vi "LoopselFF.VI"() -> ()   [LabVIEW 2015]
panel:
  in  "pos slope":u8=1
  in  "both slopes":u8
  in  "block Trig 0/1":u8
  in  "DAT in 10ns":u32
  out "FIFO overflow":bool
  in  "extTrig 0/1":u8
  in  "stop all":bool
  in  "Arm/Clear arry":bool
  in  "Slide":u32(slide)=1 scale=1.0..1000.0
  in  "frequency[Hz]":u32
  in  "no.of samples (nos)":u32=1000
  in  "exposuretime[ms]":dbl=0.02 format="%.3f"
  out "Signalverlaufgraph":u16[](graph)
  # "Abort with ESC"
  # "Start with run"
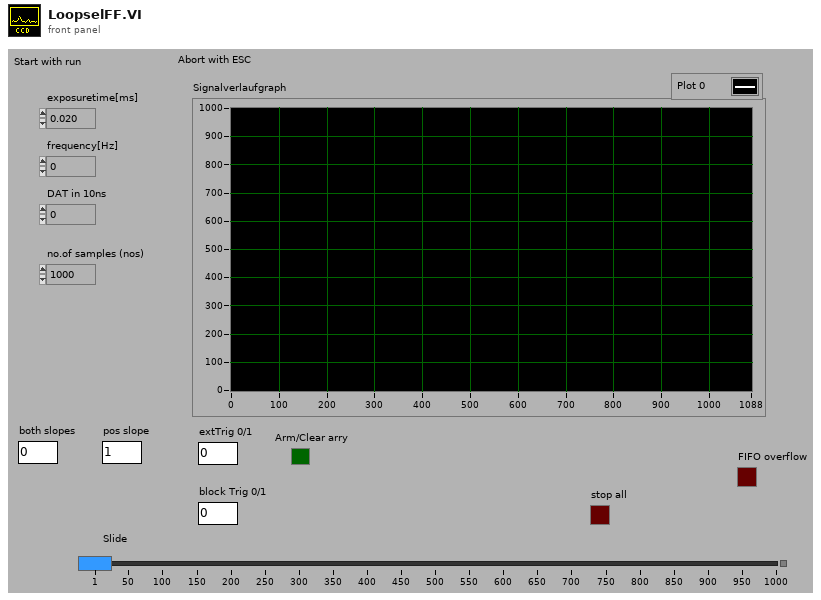
[diagram p1: front panel]
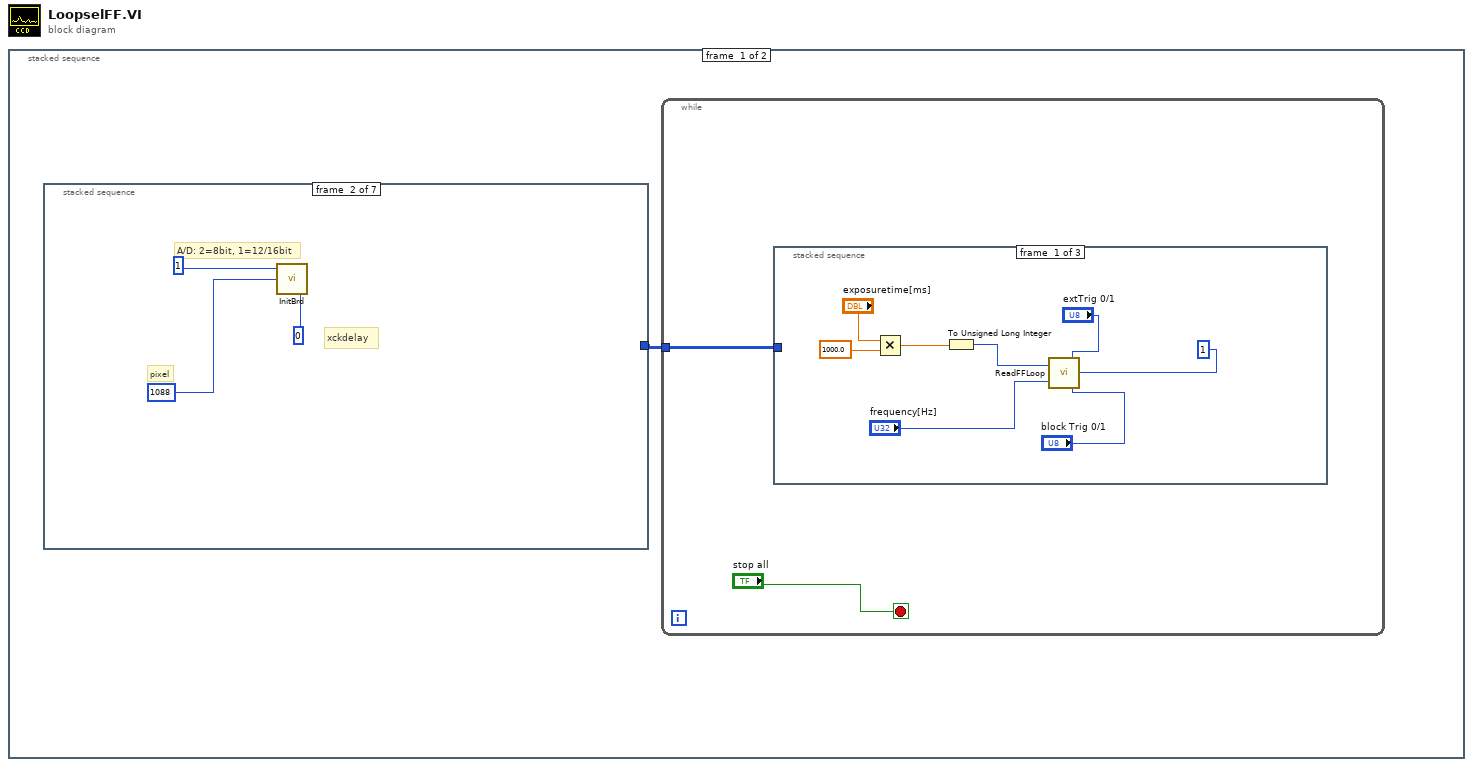
[diagram p0: block diagram]
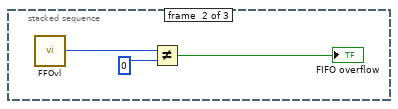
[diagram p2: hidden frame]
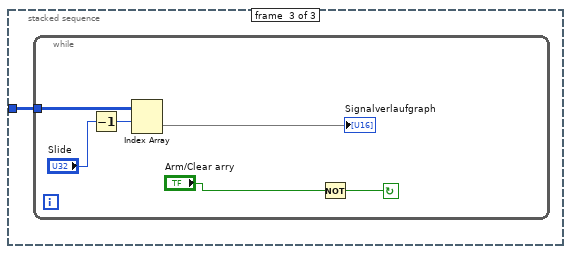
[diagram p3: hidden frame]
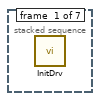
[diagram p4: hidden frame]
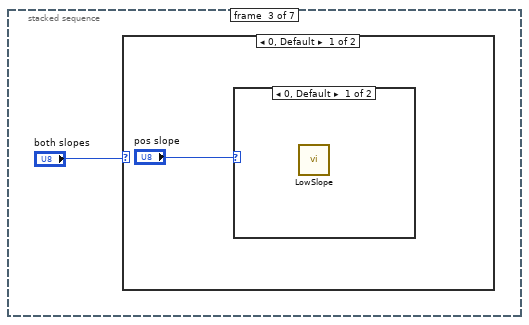
[diagram p5: hidden frame]
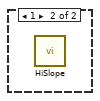
[diagram p6: hidden frame]
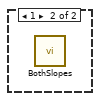
[diagram p7: hidden frame]
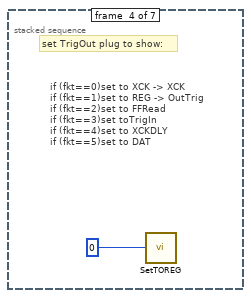
[diagram p8: hidden frame]
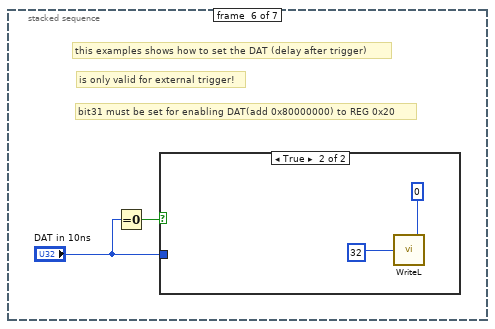
[diagram p10: hidden frame]
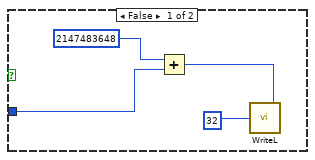
[diagram p11: hidden frame]
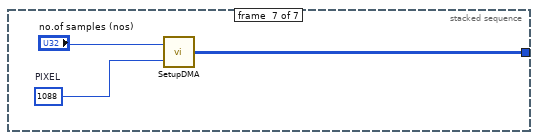
[diagram p12: hidden frame]
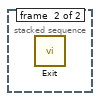
[diagram p13: hidden frame]
diagram:
  n1 = stacked-sequence {
    frame #0 {
      n2 = stacked-sequence {
        tunnel: [_ _ _ _ _ _ w38] -> w1
        frame #0 {
          n3 = call "InitDrv.vi"() -> ()  [unwired: 1 in]
        }
        frame #1 {
          # "pixel"
          # "xckdelay"
          # "A/D: 2=8bit, 1=12/16bit"
          n4 = call "InitBrd.vi"("xckdly"=u32 0, "pixel"=u32 1088, "flag816"=u32 1) -> ()  [unwired: 3 in]
        }
        frame #2 {
          n5 = case shown="0, Default" "both slopes" {
            frame 0, Default {
              n6 = case shown="0, Default" "pos slope" {
                frame 0, Default {
                  n7 = call "LowSlope.vi"() -> ()  [unwired: 1 in]
                }
                frame 1 {
                  n8 = call "HiSlope.vi"() -> ()  [unwired: 1 in]
                }
              }
            }
            frame 1 {
              n9 = call "BothSlopes.vi"() -> ()  [unwired: 1 in]
            }
          }
        }
        frame #3 {
          # "set TrigOut plug to show:"
          # "if (fkt==0)set to XCK -> XCK\nif (fkt==1)set to REG -> OutTrig\nif (fkt==2)set to FFRead\nif (fkt==3)set toTrigIn\nif (fkt==4)set to XCKDLY\nif (fkt==5)set to DAT"
          n10 = call "SetTOREG.vi"("fkt"=u8 0) -> ()
        }
        frame #4 {
        }
        frame #5 {
          # "bit31 must be set for enabling DAT(add 0x80000000) to REG 0x20"
          # "is only valid for external trigger!"
          # "this examples shows how to set the DAT (delay after trigger)"
          n11 = Equal To 0?(x="DAT in 10ns") -> (x = 0?=w29:bool)
          n12 = case shown="True" w29 {
            tunnel: "DAT in 10ns" -> [w30 _]
            frame False {
              n13 = Add(x=u32 2147483648, y=w30) -> (x+y=w33:u32)
              n14 = call "WriteL.vi"("val"=w33, "offset"=u32 32) -> ()
            }
            frame True {
              n15 = call "WriteL.vi"("val"=0, "offset"=u32 32) -> ()
            }
          }
        }
        frame #6 {
          w37 = u32 1088  # PIXEL
          n16 = call "SetupDMA.vi"("pixel"=w37, "nos"="no.of samples (nos)") -> ("Data Values"=w38:u16[][])
        }
      }
      n17 = while {
        tunnel: w1 -> [w3]
        stop <- "stop all" stop-if-true
        n18 = stacked-sequence {
          tunnel: w3 -> [_ _ w15]
          frame #0 {
            n19 = Multiply(x="exposuretime[ms]", y=1000.0) -> (x*y=w11:dbl)
            n20 = To Unsigned Long Integer(number=w11) -> (unsigned 32bit integer=w8:u32)
            n21 = call "ReadFFLoop.vi"("exptus"=w8, "freq"="frequency[Hz]", "ExtTrig"="extTrig 0/1", "btrig_ch"=u32 1, "blocktrigger"="block Trig 0/1") -> ()
          }
          frame #1 {
            n22 = call "FFOvl.vi"() -> ("FFOvl"=w13:u8)  [unwired: 1 in]
            n23 = Not Equal?(x=w13, y=0) -> (x != y?=→"FIFO overflow":bool)
          }
          frame #2 {
            n24 = while {
              tunnel: w15 -> [w19]
              stop <- w17 continue-if-true
              n25 = Decrement(x="Slide") -> (x-1=w21:u32)
              n26 = Index Array(array=w19, index (row)=w21) -> (element=→"Signalverlaufgraph":u16[])  [unwired: 1 in]
              n27 = Not(x="Arm/Clear arry") -> (.not. x?=w17:bool)
            }
          }
        }
      }
    }
    frame #1 {
      n28 = call "Exit.vi"() -> ()  [unwired: 1 in]
    }
  }
